vi "Update MWWL Range Indicator.vi"(8 "error in (no error)":errorcluster, 10 "Microwave Range":dbl, 11 "MWWL Verification in":refnum<class "MWWL Verification.lvclass">) -> (0 "error out":errorcluster, 3 "MWWL Verification out":refnum<class "MWWL Verification.lvclass">)   [LabVIEW 2017, in "MWWL Verification.lvlib" / "MWWL Verification.lvclass"]
uses:
  MWWL Verification.lvclass
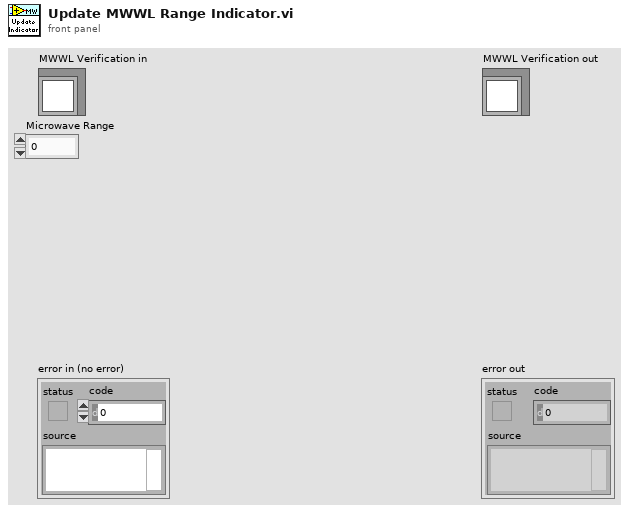
[diagram p1: front panel]
types:
  T1 = typedef "MWWL Verification.lvlib/Ranges.ctl" = cluster{"LASER A":dbl, "LASER B":dbl, "LASER C":dbl, "LASER D":dbl, "ULS":dbl, "Microwave":dbl}
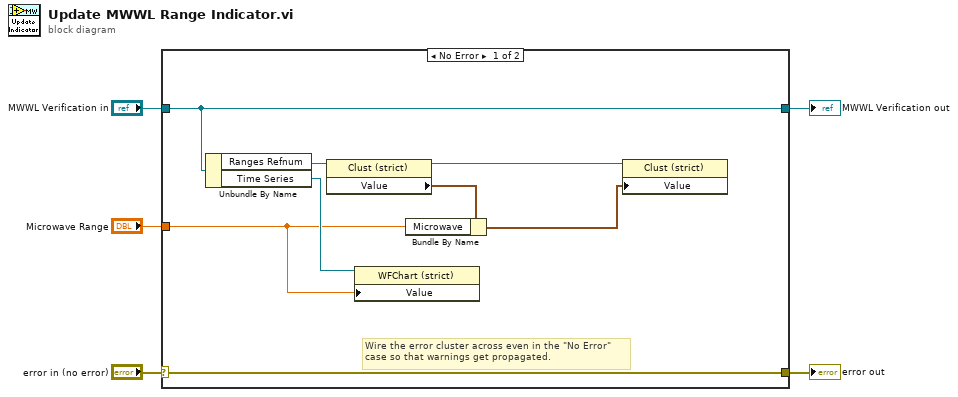
[diagram p0: block diagram]
diagram:
  n1 = case shown="No Error" "error in (no error)" {
    selector: "error in (no error)" -> [w13 w15]
    tunnel: [w13 w15] -> w4
    tunnel: [w12 w14] -> w2
    tunnel: "MWWL Verification in" -> [w12 w14]
    tunnel: "Microwave Range" -> [w6 _]
    frame No Error {
      # "Wire the error cluster across even in the \"No Error\"\ncase so that warnings get propagated."
      n2 = Unbundle By Name(w12) -> ("Ranges Refnum"=w11:refnum<vi>, "Time Series"=w7:refnum<vi>)
      n3 = property class="Clust (strict)"(reference=w11) -> (reference out=w10:refnum<vi>, "Value"=w9:T1)  [unwired: 1 in, 1 out]
      n4 = property class="WFChart (strict)"(reference=w7, "Value"=w6) -> ()  [unwired: 1 in, 2 out]
      n5 = Bundle By Name(cluster=w9, "Microwave"=w6) -> (w8:T1)
      n6 = property class="Clust (strict)"(reference=w10, "Value"=w8) -> ()  [unwired: 1 in, 2 out]
    }
    frame Error {
    }
  }
  "error out" <- w4
  "MWWL Verification out" <- w2
